vi "User Event FGV.vi"() -> (3 "User Event out":refnum<user-event>)   [LabVIEW 2018, in "Common.lvlib"]
uses:
  Common.lvlib
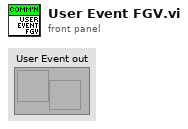
[diagram p1: front panel]
types:
  T1 = cluster{"Source":string, "Message":string, "Recipient":string, "Data":variant}
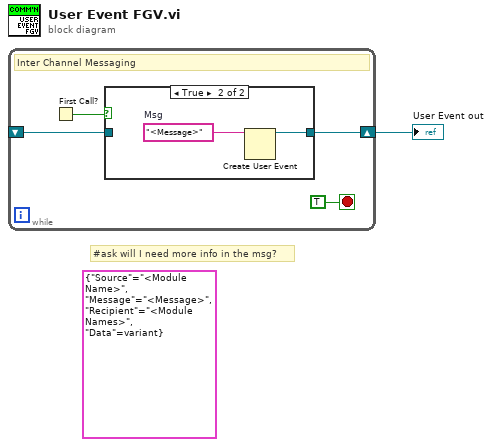
[diagram p0: block diagram]
diagram:
  (unwired) T1 {"Source"="<Module Name>", "Message"="<Message>", "Recipient"="<Module Names>", "Data"=variant}
  # "#ask will I need more info in the msg?"
  n1 = while {
    shift-right: [w4] -> w1
    shift-left: _ -> [w3]
    stop <- TRUE stop-if-true
    # "Inter Channel Messaging"
    n2 = First Call?() -> (First Call?: T/F=w5:bool)
    n3 = case shown="True" w5 {
      tunnel: [w6 w7] -> w4
      tunnel: w3 -> [w6 _]
      frame False {
      }
      frame True {
        w8 = "<Message>"  # Msg
        n4 = Create User Event(user event datatype=w8) -> (user event=w7:refnum<user-event>)  [unwired: 1 in, 1 out]
      }
    }
  }
  "User Event out" <- w1
